vi "二维码识别与检测.vi"() -> ()   [LabVIEW 2018]
uses:
  <vilib>/userdefined/High Color/IMAQdx.ctl
  <vilib>/vision/driver/NI_Vision_Acquisition_Software.lvlib
  <vilib>/vision/NI_Vision_Development_Module.lvlib
panel:
  out "Found":bool
  in  "停止":bool
  out "Data":string
  out "Image":T1(plugin-control)
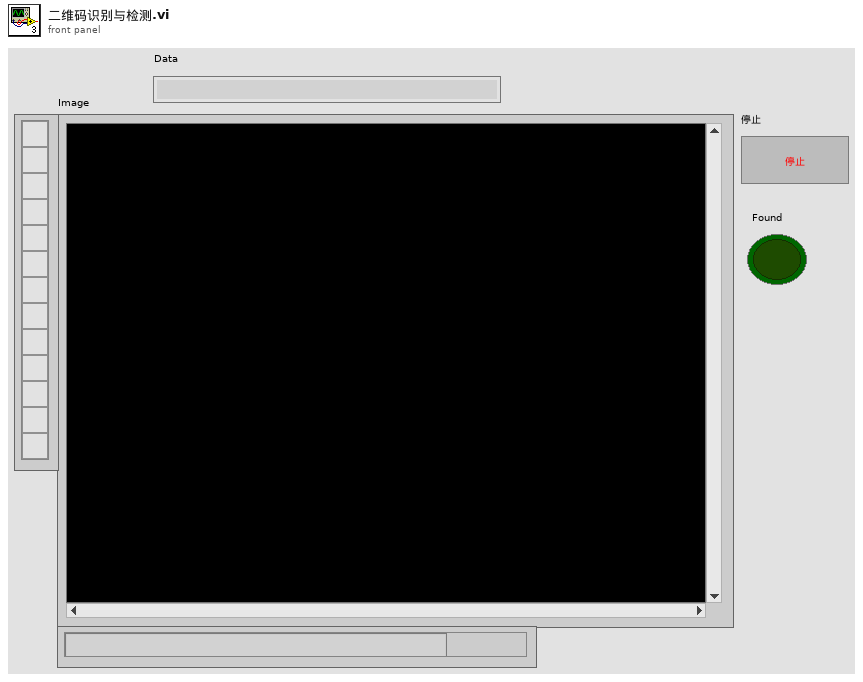
[diagram p1: front panel]
types:
  T1 = typedef "IMAQ Image.ctl" = refnum<image>
  T2 = typedef "IMAQdx.ctl" = refnum<k21>
  T3 = typedef "QR Code Report.ctl" = cluster{"Found?":bool, "Data":string, "Bounding Box":cluster{"x":sgl, "y":sgl}[], "Errors Corrected":u32, "Dimensions (Rows/Cols)":u32, "Version":u32, "QR Model":T4, "Stream Mode":T5, "Barcode Polarity":T6, "Mirrored?":bool, "Append Stream Position":u32, "Size of Append Stream":u32, "First EAN-128 ID":i32, "First Alternate Language ID":i32, "Append Stream ID":u32, "Minimum Edge Strength":u32, "Demodulation Mode":T7, "Cell Sample Size":T8, "Cell Filter Mode":T9}
  T4 = typedef "QR Code Model Type.ctl" = i32
  T5 = typedef "QR Code Stream Mode Type.ctl" = i32
  T6 = typedef "Data Matrix Polarity.ctl" = i32
  T7 = typedef "Demodulation Mode.ctl" = i32
  T8 = typedef "Cell Sample Size.ctl" = i32
  T9 = typedef "Cell Filter Mode.ctl" = i32
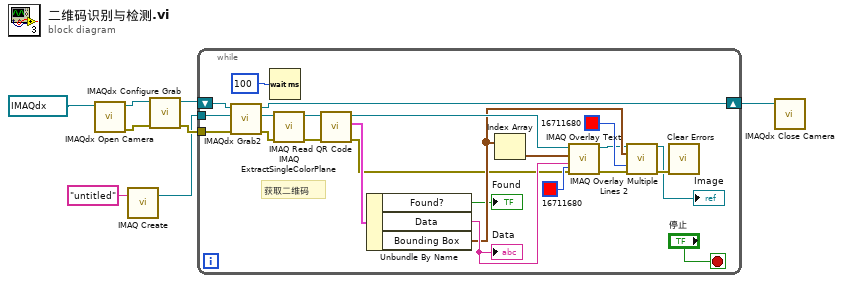
[diagram p0: block diagram]
diagram:
  n1 = call <vilib>:"IMAQdx Open Camera.vi"("Session In"=T2 "cam0") -> ("error out"=w6:errorcluster, "Session Out"=w8:T2)  [unwired: 9 in]
  n2 = call "IMAQ Create"("Image Name"="untitled") -> ("New Image"=w2:T1)  [unwired: 4 in, 1 out]
  n3 = call <vilib>:"IMAQdx Configure Grab.vi"("error in"=w6, "Session In"=w8) -> ("error out"=w5:errorcluster, "Session Out"=w7:T2)  [unwired: 8 in]
  n4 = while {
    tunnel: w5 -> [w30]
    shift-right: [w29] -> w4
    shift-left: w7 -> [w31]
    tunnel: w2 -> [w27]
    stop <- "停止" stop-if-true
    # "获取二维码"
    n5 = call <vilib>:"IMAQdx Grab2.vi"("error in"=w30, "Image In"=w27, "Session In"=w31) -> ("error out"=w11:errorcluster, "Image Out"=w25:T1, "Session Out"=w29:T2)  [unwired: 5 in, 1 out]
    n6 = Wait (ms)(milliseconds to wait=u32 100 ("等待时间（毫秒）")) -> ()  [unwired: 1 out]
    n7 = call "IMAQ ExtractSingleColorPlane"("error in (no error)"=w11, "Image Src"=w25) -> ("error out"=w12:errorcluster, "Image Dst Out"=w24:T1)  [unwired: 8 in]
    n8 = call "IMAQ Read QR Code"("error in (no error)"=w12, "Image"=w24) -> ("error out"=w13:errorcluster, "QR Code Report"=w23:T3, "Image (duplicate)"=w22:T1)  [unwired: 6 in, 1 out]
    n9 = Unbundle By Name(w23) -> ("Found?"=→"Found":bool, "Data"=w20:string, "Bounding Box"=w18:cluster{"x":sgl, "y":sgl}[])
    "Data" <- w20
    n10 = Index Array(array=w18) -> (element=w21:cluster{"x":sgl, "y":sgl})  [unwired: 1 in]
    n11 = call "IMAQ Overlay Text"("Text Color (black)"=u32 16711680, "error in (no error)"=w13, "String"=w20, "Origin"=w21, "Image"=w22) -> ("error out"=w15:errorcluster, "Image Out"=w10:T1)  [unwired: 5 in]
    n12 = call "IMAQ Overlay Multiple Lines 2"("Image"=w10, "Line End Points"=w18, "Color"=u32 16711680, "error in (no error)"=w15) -> ("Image Out"=→"Image":T1, "error out"=w14:errorcluster)  [unwired: 10 in]
    n13 = call <vilib>:"Clear Errors.vi"("error in (no error)"=w14) -> ()  [unwired: 5 in, 2 out]
  }
  n14 = call <vilib>:"IMAQdx Close Camera.vi"("Session In"=w4) -> ()  [unwired: 10 in, 1 out]
